vi "cblas dsyr.vi"(0 "x":dbl[](array[numeric]), 1 "A":T1, 3 "alpha":dbl=1.0, 5 "order":T3=101 items=["CblasRowMajor"=101, "CblasColMajor"=102], 7 "uplo":T2=121 items=["CblasUpper"=121, "CblasLower"=122], 8 "lda":i32, 10 "incx":i32=1, 11 "n":i32=-1) -> (14 "dsyr":T1, 19 "error":i32)   [LabVIEW 2017, in "NI_AALBLAS.lvlib"]
uses:
  NI_AALBLAS.lvlib
  RealMatrix.ctl
  Order.ctl
  UpLo.ctl
  <resource>/lvblas.dll
  NI_Matrix.lvlib
panel:
  # "void cblas_dsyr(order, uplo, n, alpha, *x, incx, *A, lda)"
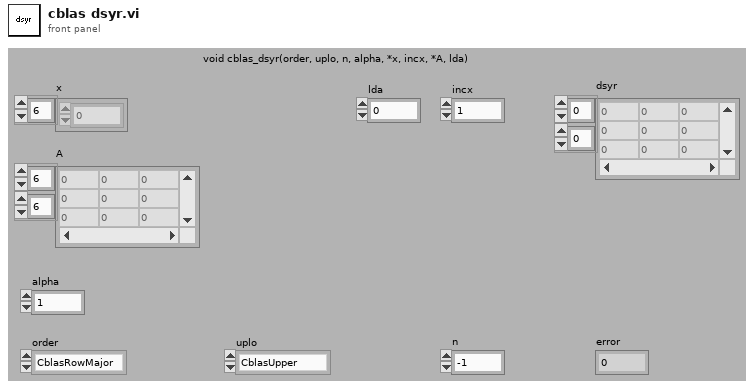
[diagram p1: front panel]
types:
  T1 = typedef "NI_Matrix.lvlib/RealMatrix.ctl" = dbl[][]
  T2 = typedef "NI_AALBLAS.lvlib/UpLo.ctl" = i32
  T3 = typedef "NI_AALBLAS.lvlib/Order.ctl" = i32
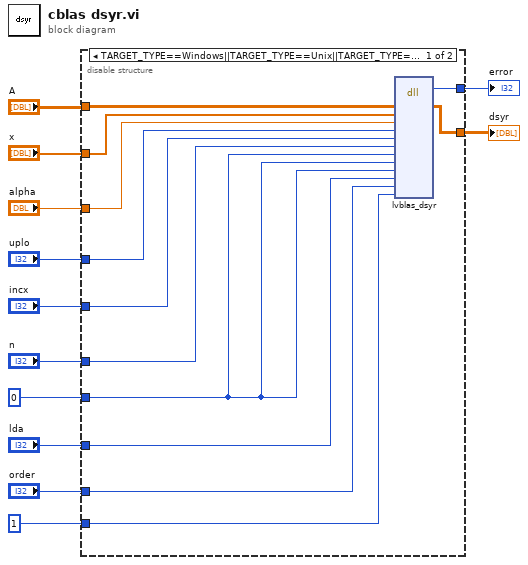
[diagram p0: block diagram]
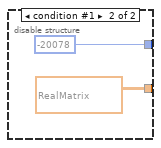
[diagram p2: hidden frame]
diagram:
  n1 = disable-structure shown="TARGET_TYPE==Windows||TARGET_TYPE==Unix||TARGET_TYPE==Mac||TARGET_TYPE==RT" {
    disable-tunnel: "x" -> [w24 _]
    disable-tunnel: "A" -> [w23 _]
    disable-tunnel: [w22 -20078 ("error")] -> w5
    disable-tunnel: 0 -> [w16 _]
    disable-tunnel: "lda" -> [w15 _]
    disable-tunnel: [w21 T1 [[0.0, 0.0, 0.0, 0.0, 0.0, 0.0, 0.0, 0.0, 0.0], [0.0, 0.0, 0.0, 0.0, 0.0, 0.0, 0.0, 0.0, 0.0], [0.0, 0.0, 0.0, 0.0, 0.0, 0.0, 0.0, 0.0, 0.0], [0.0, 0.0, 0.0, 0.0, 0.0, 0.0, 0.0, 0.0, 0.0], [0.0, 0.0, 0.0, 0.0, 0.0, 0.0, 0.0, 0.0, 0.0], [0.0, 0.0, 0.0, 0.0, 0.0, 0.0, 0.0, 0.0, 0.0], [0.0, 0.0, 0.0, 0.0, 0.0, 0.0, 1.0, 0.0, 0.0], [0.0, 0.0, 0.0, 0.0, 0.0, 0.0, 0.0, 0.0, 0.0], [0.0, 0.0, 0.0, 0.0, 0.0, 0.0, 0.0, 0.0, 4.0]] ("dsyr 2")] -> w1
    disable-tunnel: "uplo" -> [w19 _]
    disable-tunnel: "incx" -> [w18 _]
    disable-tunnel: "n" -> [w17 _]
    disable-tunnel: "alpha" -> [w20 _]
    disable-tunnel: "order" -> [w14 _]
    disable-tunnel: 1 -> [w13 _]
    frame condition #0 (active) {
      n2 = dll-call lib="C:/Program Files (x86)/National Instruments/LabVIEW 2017/resource/lvblas.*" fn="lvblas_dsyr" ("CBLAS.dll:MtrxxVectH")("a"=w23, "x"=w24, "alpha"=w20, "uplo"=w19, "IncX"=w18, "n"=w17, "startARow"=w16, "startACol"=w16, "startX"=w16, "lda"=w15, "order"=w14, "check"=w13) -> ("error"=w22:i32, "a"=w21:dbl[][])  [unwired: 14 in, 2 out]
    }
    frame condition #1 {
    }
  }
  "error" <- w5
  "dsyr" <- w1
